vi "GV_GetPresetSaveSettings.vi"(8 "error in (no error)":errorcluster, 11 "Gviewer in":refnum<class "Gviewer.lvclass">) -> (0 "error out":errorcluster, 2 "PresetSaveSettings":T1, 3 "Gviewer out":refnum<class "Gviewer.lvclass">)   [LabVIEW 2020, in "Sgraph_lib_V1.lvlib" / "Gviewer.lvclass"]
doc: "Andre Koelewijn, 8 mar 2022\n\nGet Presets to save from class attributes"
uses:
  Gviewer.lvclass
  GV_Typedef_PresetSaveSettings.ctl
  controls/Typedef_Live.ctl
  controls/Typedef_Autoscale.ctl
  controls/LegendSet.ctl
  <vilib>/Utility/miscctls.llb/LVPositionTypeDef.ctl
  <vilib>/Utility/miscctls.llb/LVBoundsTypeDef.ctl
  controls/YgraphDef.ctl
  controls/AutoScale.ctl
  controls/MinMax.ctl
  controls/TD_Lscale.ctl
  controls/TD_Rscale.ctl
  Gviewer.lvclass/Gviewer.ctl
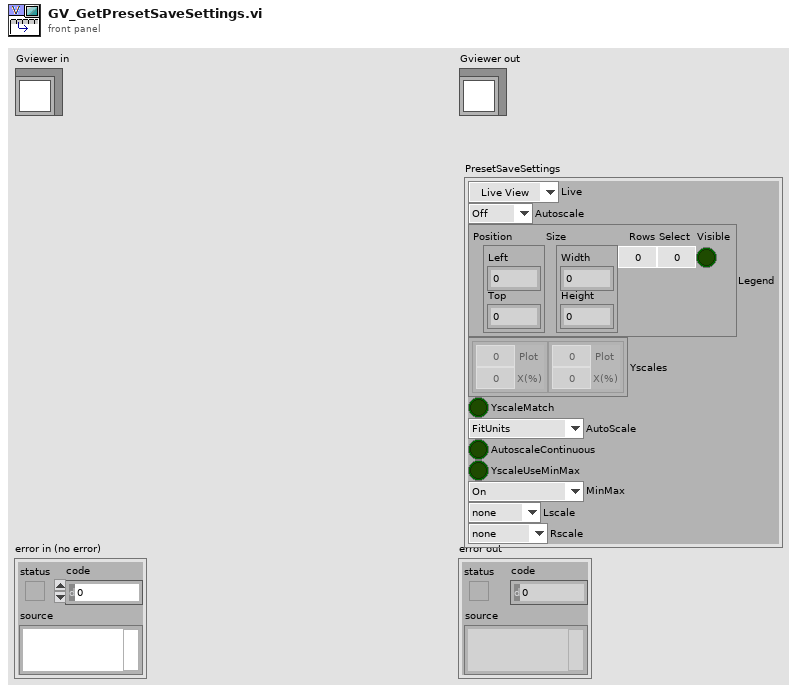
[diagram p1: front panel]
types:
  T1 = typedef "Sgraph_lib_V1.lvlib/Gviewer.lvclass/GV_Typedef_PresetSaveSettings.ctl" = cluster{"Live":T2, "Autoscale":T3, "Legend":T4, "Yscales":T7[], "YscaleMatch":bool, "AutoScale":T8, "AutoscaleContinuous":bool, "YscaleUseMinMax":bool, "MinMax":T9, "Lscale":T10, "Rscale":T11}
  T2 = typedef "Sgraph_lib_V1.lvlib/Gviewer.lvclass/Typedef_Live.ctl" = enum16{"Live View", "Freeze"}
  T3 = typedef "Sgraph_lib_V1.lvlib/Gviewer.lvclass/Typedef_Autoscale.ctl" = enum16{"Off", "Max", "Stack", "Norm"}
  T4 = typedef "Sgraph_lib_V1.lvlib/Gviewer.lvclass/LegendSet.ctl" = cluster{"Position":T5, "Size":T6, "Rows":u32, "Select":i32, "Visible":bool}
  T5 = typedef "LVPositionTypeDef.ctl" = cluster{"Left":i32, "Top":i32}
  T6 = typedef "LVBoundsTypeDef.ctl" = cluster{"Width":u32, "Height":u32}
  T7 = typedef "Sgraph_lib_V1.lvlib/Gviewer.lvclass/YgraphDef.ctl" = cluster{"Plot":i32, "X(%)":dbl}
  T8 = typedef "Sgraph_lib_V1.lvlib/Gviewer.lvclass/AutoScale.ctl" = enum16{"FitUnits", "FitAnalogs", "FitAll", "Stack"}
  T9 = typedef "Sgraph_lib_V1.lvlib/Gviewer.lvclass/MinMax.ctl" = enum16{"On", "Off", "Focus"}
  T10 = typedef "Sgraph_lib_V1.lvlib/Gviewer.lvclass/TD_Lscale.ctl" = enum16{"none", "one", "many"}
  T11 = typedef "Sgraph_lib_V1.lvlib/Gviewer.lvclass/TD_Rscale.ctl" = enum16{"none", "one", "all"}
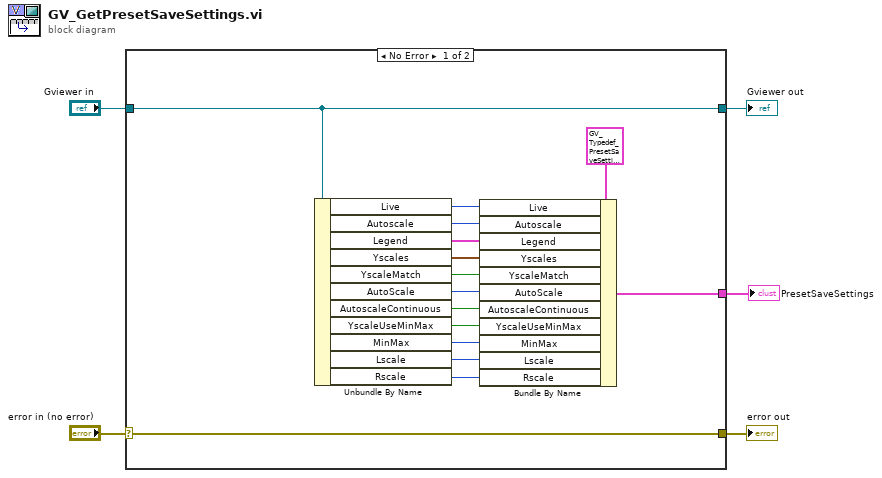
[diagram p0: block diagram]
diagram:
  n1 = case shown="No Error" "error in (no error)" {
    selector: "error in (no error)" -> [w20 w22]
    tunnel: [w20 w22] -> w4
    tunnel: [w17 w21] -> w2
    tunnel: "Gviewer in" -> [w17 w21]
    tunnel: [w18 _] -> w1
    frame No Error {
      n2 = Unbundle By Name(w17) -> ("Live"=w16:T2, "Autoscale"=w15:T3, "Legend"=w14:T4, "Yscales"=w13:T7[], "YscaleMatch"=w12:bool, "AutoScale"=w11:T8, "AutoscaleContinuous"=w10:bool, "YscaleUseMinMax"=w9:bool, "MinMax"=w8:T9, "Lscale"=w7:T10, "Rscale"=w6:T11)
      n3 = Bundle By Name(cluster=T1 {"Live"=enum."Live View", "Autoscale"=enum."Off", "Legend"={"Position"={"Left"=0, "Top"=0}, "Size"={"Width"=0, "Height"=0}, "Rows"=0, "Select"=0, "Visible"=FALSE}, "Yscales"=[], "YscaleMatch"=FALSE, "AutoScale"=enum."FitUnits", "AutoscaleContinuous"=FALSE, "YscaleUseMinMax"=FALSE, "MinMax"=enum."On", "Lscale"=enum."none", "Rscale"=enum."none"} ("PresetSaveSettings"), "Live"=w16, "Autoscale"=w15, "Legend"=w14, "Yscales"=w13, "YscaleMatch"=w12, "AutoScale"=w11, "AutoscaleContinuous"=w10, "YscaleUseMinMax"=w9, "MinMax"=w8, "Lscale"=w7, "Rscale"=w6) -> (w18:T1)
    }
    frame Error {
    }
  }
  "error out" <- w4
  "Gviewer out" <- w2
  "PresetSaveSettings" <- w1
